vi "Connect Error Terminals.vi"(8 "error in (no error)":errorcluster, 9 "error controls in":cluster{"in":refnum<vi>, "out":refnum<vi>}, 10 "case structure in":refnum<vi>, 11 "VI in":refnum<vi>) -> (0 "error out":errorcluster, 1 "error controls out":cluster{"in":refnum<vi>, "out":refnum<vi>}, 2 "case structure out":refnum<vi>, 3 "VI out":refnum<vi>, 4 "error terminals":cluster{"in":refnum<vi>, "out":refnum<vi>}, 6 "error case tunnels":cluster{"in":refnum<vi>, "out":refnum<vi>})   [LabVIEW 2017]
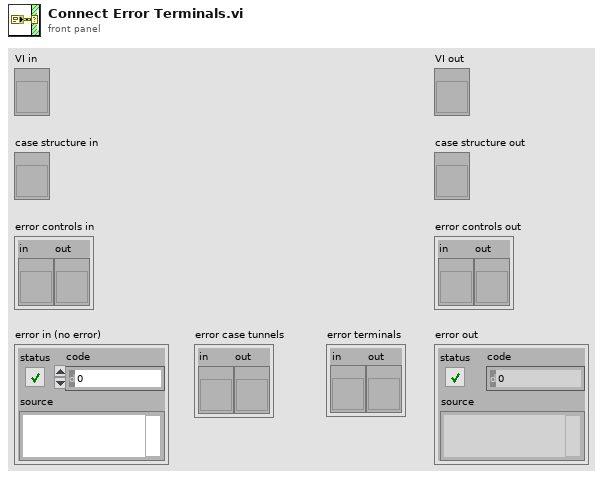
[diagram p1: front panel]
types:
  T1 = enum32{"Top Edges", "Vertical Centers", "Bottom Edges", "Left Edges", "Horizontal Centers", "Right Edges"}
  T2 = cluster{"Terminal":refnum<vi>, "Terminal":refnum<vi>}
  T3 = cluster{"Selector":refnum<vi>, "new tunnel":refnum<vi>}
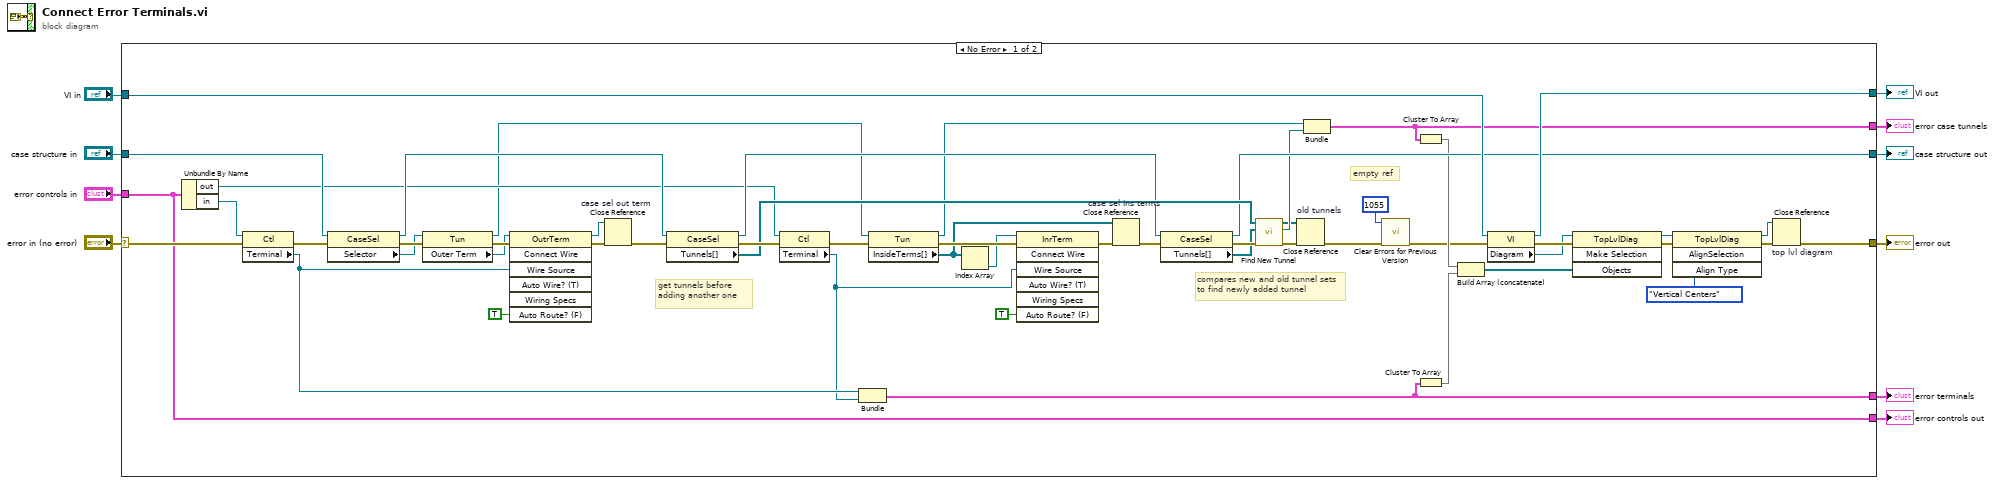
[diagram p0: block diagram]
diagram:
  n1 = case shown="No Error" "error in (no error)" {
    selector: "error in (no error)" -> [w24 w64]
    tunnel: "case structure in" -> [w50 w66]
    tunnel: "error controls in" -> [w23 w65]
    tunnel: [w18 _] -> w8
    tunnel: [w23 w65] -> w7
    tunnel: [w35 w64] -> w6
    tunnel: "VI in" -> [w33 w67]
    tunnel: [w32 w67] -> w4
    tunnel: [w27 w66] -> w3
    tunnel: [w17 _] -> w2
    frame No Error {
      # "empty ref"
      # "compares new and old tunnel sets to find newly added tunnel"
      # "get tunnels before adding another one"
      n2 = Unbundle By Name(w23) -> ("out"=w31:refnum<vi>, "in"=w46:refnum<vi>)
      n3 = property class="Ctl"(reference=w46, error in=w24) -> (error out=w53:errorcluster, "Terminal"=w20:refnum<vi>)  [unwired: 1 out]
      n4 = property class="CaseSel"(reference=w50, error in=w53) -> (reference out=w54:refnum<vi>, error out=w52:errorcluster, "Selector"=w49:refnum<vi>)
      n5 = property class="Tun"(reference=w49, error in=w52) -> (reference out=w30:refnum<vi>, error out=w51:errorcluster, "Outer Term"=w47:refnum<vi>)
      n6 = invoke class="OutrTerm" method="Connect Wire"(reference=w47, error in=w51, "Wire Source"=w20, "Auto Route? (F)"=TRUE) -> (reference out=w42:refnum<vi>, error out=w44:errorcluster)  [unwired: 3 in, 5 out]
      n7 = Close Reference "case sel out term"(reference=w42, error in (no error)=w44) -> (error out=w43:errorcluster)
      n8 = property class="CaseSel"(reference=w54, error in=w43) -> (reference out=w55:refnum<vi>, error out=w59:errorcluster, "Tunnels[]"=w56:refnum<vi>[])
      n9 = property class="Ctl"(reference=w31, error in=w59) -> (error out=w58:errorcluster, "Terminal"=w19:refnum<vi>)  [unwired: 1 out]
      n10 = Bundle("Terminal"=w20, "Terminal"=w19) -> (w18:T2)  [unwired: 1 in]
      n11 = property class="Tun"(reference=w30, error in=w58) -> (reference out=w29:refnum<vi>, error out=w60:errorcluster, "InsideTerms[]"=w28:refnum<vi>[])
      n12 = Index Array(array=w28) -> (element=w48:refnum<vi>)  [unwired: 1 in]
      n13 = invoke class="InrTerm" method="Connect Wire"(reference=w48, error in=w60, "Wire Source"=w19, "Auto Route? (F)"=TRUE) -> (error out=w45:errorcluster)  [unwired: 3 in, 6 out]
      n14 = Close Reference "case sel ins terms"(reference=w28, error in (no error)=w45) -> (error out=w41:errorcluster)
      n15 = property class="CaseSel"(reference=w55, error in=w41) -> (reference out=w27:refnum<vi>, error out=w63:errorcluster, "Tunnels[]"=w57:refnum<vi>[])
      n16 = call "Find New Tunnel.vi"("error in (no error)"=w63, "new tunnels in"=w57, "old tunnels in"=w56) -> ("error out"=w61:errorcluster, "new tunnel"=w26:refnum<vi>, "old tunnels out"=w25:refnum<vi>[])  [unwired: 6 in]
      n17 = Close Reference "old tunnels"(reference=w25, error in (no error)=w61) -> (error out=w13:errorcluster)
      n18 = Bundle("Selector"=w29, "new tunnel"=w26) -> (w17:T3)  [unwired: 1 in]
      n19 = call "Clear Errors for Previous Version.vi"("error in (no error)"=w13, "code"=1055) -> ("error out"=w12:errorcluster)  [unwired: 9 in]
      n20 = Cluster To Array(cluster=w17) -> (array=w14:refnum<vi>[])
      n21 = Cluster To Array(cluster=w18) -> (array=w16:refnum<vi>[])
      n22 = Build Array (concatenate)(w14, w16) -> (w15:refnum<vi>[])
      n23 = property class="VI"(reference=w33, error in=w12) -> (reference out=w32:refnum<vi>, error out=w62:errorcluster, "Diagram"=w36:refnum<vi>)
      n24 = invoke class="TopLvlDiag" method="Make Selection"(reference=w36, error in=w62, "Objects"=w15) -> (reference out=w40:refnum<vi>, error out=w38:errorcluster)  [unwired: 1 in, 2 out]
      n25 = invoke class="TopLvlDiag" method="AlignSelection"(reference=w40, error in=w38, "Align Type"=T1."Vertical Centers") -> (reference out=w34:refnum<vi>, error out=w37:errorcluster)  [unwired: 1 in, 2 out]
      n26 = Close Reference "top lvl diagram"(reference=w34, error in (no error)=w37) -> (error out=w35:errorcluster)
    }
    frame Error {
    }
  }
  "error out" <- w6
  "case structure out" <- w3
  "error controls out" <- w7
  "error case tunnels" <- w2
  "error terminals" <- w8
  "VI out" <- w4
